vi "Main Tclk.vi"() -> ()   [LabVIEW 2018] (continued)
                w6374 = sgl 0.0 ("Single")
                n1042 = shared-variable ".\\Zeiss Library.lvlib\\Milling Z Voltage"() -> (w6355:sgl)  [unwired: 1 in, 1 out]
                "Milling Z voltage (V)" <- w6355
                n1043 = local read "FIB Options"() -> (w6358:T33)
                n1044 = local read "FIB Scan Parameters"() -> (w6356:T32)
                n1045 = local read "Milling para"() -> (w6354:T35)
                n1046 = Unbundle By Name(w6358) -> ("Flip z"=w6373:bool)
                n1047 = Unbundle By Name(w6354) -> ("FIB FOV (um)"=w6366:sgl)
                n1048 = Unbundle By Name(w6354) -> ("X size (um)"=w6352:sgl, "Line milling time (s)"=w6350:sgl, "Lines auto pause"=w6349:u16)
                n1049 = Unbundle By Name(w6356) -> ("Z size (V)"=w6357:dbl)
                n1050 = Negate(x=w6355) -> (-x=w6359:sgl)
                n1051 = Select(t=w6359, s=w6373, f=w6355) -> (s? t:f=w6360:sgl)
                n1052 = Negate(x=w6374) -> (-x=w6375:sgl)
                n1053 = Divide(x=w6360, y=w6357) -> (x/y=w6361:dbl)
                n1054 = Select(t=w6374, s=w6373, f=w6375) -> (s? t:f=w6377:sgl)
                n1055 = Multiply(x=w6361, y=w6366) -> (x*y=w6376:dbl)
                n1056 = Add(x=w6377, y=w6376) -> (x+y=w6378:dbl)
                "FIB profile Y center (um)" <- w6378
                n1057 = call "Milling parameter to trapezoidal shape.vi"("Y location (um)"=w6378, "Milling para"=w6354) -> ("X end"=w6371:dbl, "X start"=w6370:dbl, "X size (um) @ Y"=w6353:dbl)  [unwired: 5 in, 2 out]
                n1058 = expression code="x/2"(w6366) -> (w6367:sgl)
                n1059 = Add(x=w6370, y=w6371) -> (x+y=w6365:dbl)
                n1060 = Divide(x=w6353, y=w6352) -> (x/y=w6351:dbl)
                n1061 = expression code="x/2-30"(w6353) -> (w6363:dbl)
                n1062 = expression code="x/2"(w6365) -> (w6368:dbl)
                n1063 = Compound Arithmetic op=MULTIPLY(w6351, w6350, w6349) -> (→"Milling time (s)":dbl)
                n1064 = Random Number (0-1)() -> (number: 0 to 1=w6362:dbl)
                n1065 = Random Number (0-1)() -> (number: 0 to 1=w6344:dbl)
                n1066 = expression code="(x*2-1)*10"(w6362) -> (w6347:dbl)
                n1067 = Multiply(x=w6367, y=w6368) -> (x*y=w6369:dbl)
                n1068 = In Range and Coerce(upper limit=w6367, x=w6363, lower limit=0.0) -> (coerced(x)=w6346:dbl)  [unwired: 1 out]
                n1069 = Greater?(x=0.5, y=w6344) -> (0:w6342:bool)
                n1070 = Add(x=w6347, y=w6346) -> (x+y=w6345:dbl)
                n1071 = Select(t=1.0 ("f"), s=w6342, f=-1.0) -> (s? t:f=w6339:dbl)
                n1072 = Multiply(x=w6339, y=w6345) -> (x*y=w6338:dbl)
                n1073 = Add(x=w6338, y=w6369) -> (x+y=→"FIB profile X center (um)":dbl)
              }
              frame #9 {
                n1074 = local read "Re-engage counts"() -> (w6387:u8)
                n1075 = local read "Last re-engage count"() -> (w6386:u8)
                n1076 = local read "Low Mag SEM"() -> (w6395:T30)
                n1077 = local read "FIB slice #"() -> (w6393:u32)
                n1078 = local read "Milling para"() -> (w6394:T35)
                n1079 = Unbundle By Name(w6395) -> ("Low mag scan"=w6398:bool, "Prior to main scan"=w6391:bool, "Low mag interval"=w6397:u32)
                n1080 = Select(t=u32 0, s=w6391, f=u32 1 ("t")) -> (s? t:f=w6390:u32)
                n1081 = Unbundle By Name(w6394) -> ("Auto Profile"=w6379:bool)
                n1082 = Subtract(x=w6393, y=w6390) -> (x-y=w6392:u32)
                n1083 = Equal?(x=w6387, y=w6386) -> (x = y?=w6384:bool)
                n1084 = Not Equal To 0?(x=w6386) -> (x != 0?=w6385:bool)
                n1085 = Quotient & Remainder(x=w6392, y=w6397) -> (x-y*floor(x/y)=w6400:u32)  [unwired: 1 out]
                n1086 = And(x=w6384, y=w6385) -> (x .and. y?=w6382:bool)
                n1087 = local read "FIB"() -> (w6396:bool)
                n1088 = Equal To 0?(x=w6400) -> (x = 0?=w6399:bool)
                n1089 = Compound Arithmetic op=AND(w6396, w6398, w6399) -> (w6383:bool)
                n1090 = Or(x=w6382, y=w6383) -> (x .or. y?=w6381:bool)
                n1091 = And(x=w6381, y=w6379) -> (x .and. y?=w6380:bool)
                n1092 = case shown="False" w6380 {
                  frame False {
                  }
                  frame True {
                    n1093 = stacked-sequence {
                      frame #0 {
                        n1094 = local write "FIB Profile"(TRUE ("FIB Profile")) -> ()
                        n1095 = local write "Enable logging"(FALSE ("Enable logging")) -> ()
                        n1096 = Wait (ms)(milliseconds to wait=u32 200) -> ()  [unwired: 1 out]
                      }
                      frame #1 {
                        n1097 = local read "Machine Type"() -> (w6404:u8)
                        n1098 = case shown="2" w6404 {
                          frame 0, Default {
                            w6406 = sgl 90.0 ("UL-Ang")
                            n1099 = local read "FIB profile X center (um)"() -> (w6408:dbl)
                            n1100 = local read "FIB profile Y center (um)"() -> (w6409:dbl)
                            n1101 = local read "HV Data Output"() -> (w6407:T18)
                            n1102 = local read "FIB HW Config"() -> (w6416:T23)
                            n1103 = local read "FIB Options"() -> (w6417:T33)
                            n1104 = local read "Milling para"() -> (w6413:T35)
                            n1105 = local read "FIB Scan Parameters"() -> (w6414:T32)
                            n1106 = local read "Parameter Names"() -> (w6420:string[])
                            n1107 = Bundle By Name(cluster=w6414, "Frame line rampdown ratio"=0.0, "Oversampling"=u16 5) -> (w6418:T32)
                            n1108 = Bundle By Name(cluster=w6413, "X size (um)"=sgl 0.1, "Z size (um)"=sgl 10.0 ("Y size (um)"), "X center (um)"=w6408, "Z center (um)"=w6409, "UL-Ang"=w6406, "UR-Ang"=w6406) -> (w6412:T35)
                            n1109 = local read "Active logging channels"() -> (w6419:string)
                            n1110 = local write "Status message"("Scanning FIB vertically to obtain beam profile" ("Status message")) -> ()
                            n1111 = local read "Api"() -> (w6405:refnum<k7>)
                            n1112 = call "FIB profile.vi"("ActiveX Container"=w6405, "HV Data Output"=w6407, "Parameter Names"=w6420, "Active logging channels"=w6419, "Scan Para"=w6418, "Milling para"=w6412, "Options"=w6417, "HW Config"=w6416) -> ("Measurements"=w6422:dbl[][])  [unwired: 1 in, 2 out]
                            n1113 = local write "Measurements"(w6422) -> ()
                          }
                          frame 2 {
                            w6425 = sgl 90.0 ("UL-Ang")
                            n1114 = local read "FIB profile X center (um)"() -> (w6427:dbl)
                            n1115 = local read "FIB profile Y center (um)"() -> (w6428:dbl)
                            n1116 = local read "FIB HW Config"() -> (w6435:T23)
                            n1117 = local read "FIB Options"() -> (w6436:T33)
                            n1118 = local read "Milling para"() -> (w6432:T35)
                            n1119 = local read "FIB Scan Parameters"() -> (w6433:T32)
                            n1120 = local read "Parameter Names"() -> (w6439:string[])
                            n1121 = local read "Capella HV Data Output"() -> (w6426:T17)
                            n1122 = Bundle By Name(cluster=w6433, "Frame line rampdown ratio"=0.0, "Oversampling"=u16 5) -> (w6437:T32)
                            n1123 = local read "Active logging channels"() -> (w6438:string)
                            n1124 = Bundle By Name(cluster=w6432, "X size (um)"=sgl 0.1, "Z size (um)"=sgl 10.0 ("Y size (um)"), "X center (um)"=w6427, "Z center (um)"=w6428, "UL-Ang"=w6425, "UR-Ang"=w6425) -> (w6431:T35)
                            n1125 = local write "Status message"("Scanning FIB vertically to obtain beam profile" ("Status message")) -> ()
                            n1126 = local read "Api"() -> (w6424:refnum<k7>)
                            n1127 = call "FIB profile.vi"("ActiveX Container"=w6424, "Capella HV Data Output"=w6426, "Parameter Names"=w6439, "Active logging channels"=w6438, "Scan Para"=w6437, "Milling para"=w6431, "Options"=w6436, "HW Config"=w6435) -> ("Measurements"=w6441:dbl[][])  [unwired: 1 in, 2 out]
                            n1128 = local write "Measurements"(w6441) -> ()
                          }
                        }
                      }
                      frame #2 {
                        n1129 = local write "FIB Profile"(FALSE ("FIB Profile")) -> ()
                        n1130 = local write "Enable logging"(TRUE ("Enable logging")) -> ()
                      }
                    }
                  }
                }
              }
              frame #10 {
                n1131 = local read "FIB"() -> (w6445:bool)
                n1132 = case shown="True" w6445 {
                  frame False {
                  }
                  frame True {
                    n1133 = local read "Hardware Configuration"() -> (w6453:T25)
                    n1134 = Unbundle By Name(w6453) -> ("Shutter Drive"=w6452:tag)
                    n1135 = local read "Damping"() -> (w6446:bool)
                    n1136 = call "Shutter Swing V3.vi"("Shutter Drive"=w6452, "Damping"=w6446, "Shutter close"=FALSE) -> ("Shutter close fdbk"=w6449:bool, "Fail #"=w6447:u8, "SEM shutter status"=w6450:string)  [unwired: 2 in, 4 out]
                    n1137 = Greater Than 0?(x=w6447) -> (x > 0?=→"SEM shutter failed active":bool)
                    n1138 = local write "SEM shutter status"(w6450) -> ()
                    n1139 = local write "Fail #"(w6447) -> ()
                    n1140 = local write "SEM Shutter"(w6449) -> ()
                  }
                }
              }
              frame #11 {
                n1141 = local read "Low Mag SEM"() -> (w6456:T30)
                n1142 = local read "FIB slice #"() -> (w6455:u32)
                n1143 = Unbundle By Name(w6456) -> ("Low mag scan"=w6459:bool, "Prior to main scan"=w6458:bool, "Low mag interval"=w6454:u32)
                n1144 = Quotient & Remainder(x=w6455, y=w6454) -> (x-y*floor(x/y)=w6461:u32)  [unwired: 1 out]
                n1145 = local read "FIB"() -> (w6457:bool)
                n1146 = Equal To 0?(x=w6461) -> (x = 0?=w6460:bool)
                n1147 = Compound Arithmetic op=AND(w6457, w6459, w6458, w6460) -> (w6462:bool)
                n1148 = case shown="True" w6462 {
                  frame False {
                    n1149 = local write "Low Mag SEM on"(FALSE ("Mid Mag SEM on")) -> ()
                    n1150 = local write "LM overhead"(u32 0 ("LM overhead")) -> ()
                  }
                  frame True {
                    n1151 = stacked-sequence {
                      seq-local: [w6468 _] -> [_ w6480]
                      frame #0 {
                        n1152 = local read "LM SEM scan time"() -> (w6467:dbl)
                        n1153 = local read "Tiled scan inputs"() -> (w6469:T6)
                        n1154 = local read "SEM HW Config"() -> (w6470:T9)
                        n1155 = local read "Detector Information"() -> (w6471:T8)
                        n1156 = local read "SEM Scan Parameters"() -> (w6472:T26)
                        n1157 = local read "SEM Options"() -> (w6473:T27)
                        n1158 = local read "Focus Index Options"() -> (w6465:T28)
                        n1159 = local read "File Information"() -> (w6474:T31)
                        n1160 = local read "Milling para"() -> (w6475:T35)
                        n1161 = Bundle By Name(cluster=w6469, "HW Config"=w6470, "Det Info"=w6471, "SEM Scan Parameters"=w6472, "SEM Options"=w6473, "Focus Index Options"=w6465, "File Information"=w6474, "Milling para"=w6475) -> (w6468:T6)
                        n1162 = expression code="x+10"(w6467) -> (w6466:dbl)
                        n1163 = local write "LM overhead"(w6466) -> ()
                      }
                      frame #1 {
                        w6481 = FALSE ("GetInfo")
                        n1164 = local read "SEM Low Mag Scan Parameters"() -> (w6483:T5)
                        n1165 = local read "File Information"() -> (w6484:T31)
                        n1166 = Unbundle By Name(w6484) -> ("File path"=w6486:path)
                        n1167 = local write "Status message"("SEM Low Mag Scan" ("Status message")) -> ()
                        n1168 = Build Path(base path=w6486, name or relative path="Low Mag Scans\\") -> (appended path=w6487:path)
                        n1169 = local read "Api"() -> (w6476:refnum<k7>)
                        n1170 = Bundle By Name(cluster=w6480, "SEM Options.GetInfo"=w6481, "SEM Options.PNG only"=TRUE ("PNG only"), "SEM Options.Upload"=w6481, "SEM Scan Parameters"=w6483, "File Information.File path"=w6487) -> (w6477:T6)
                        n1171 = local read "WatchDog Mode"() -> (w6478:u16)
                        n1172 = call "2D scan tiled.vi"("WatchDog Mode"=w6478, "Tiled scan inputs"=w6477, "ActiveX Container"=w6476) -> ()  [unwired: 3 in, 6 out]
                        "Low Mag SEM on" <- TRUE ("Mid Mag SEM on")
                      }
                    }
                  }
                }
              }
              frame #12 {
                n1173 = local read "Mid Mag SEM"() -> (w6500:T29)
                n1174 = local read "FIB slice #"() -> (w6499:u32)
                n1175 = Subtract(x=w6499, y=u32 2) -> (x-y=w6490:u32)
                n1176 = Unbundle By Name(w6500) -> ("Mid mag scan"=w6497:bool, "Prior to main scan"=w6504:bool, "Mid mag interval"=w6489:u32)
                n1177 = Equal?(x=u32 1 ("y"), y=w6489) -> (x = y?=w6491:bool)
                n1178 = case shown="False" w6491 {
                  tunnel: [w6508 w6511] -> w6496
                  tunnel: [w6507 w6511] -> w6495
                  tunnel: [w6505 w6511] -> w6493
                  frame False {
                    n1179 = local read "Auto Focus"() -> (w6510:bool)
                    n1180 = local read "Auto Stig"() -> (w6509:bool)
                    n1181 = local read "Auto Align"() -> (w6506:bool)
                    n1182 = Not(x=w6510) -> (.not. x?=w6507:bool)
                    n1183 = Not(x=w6509) -> (.not. x?=w6508:bool)
                    n1184 = Not(x=w6506) -> (.not. x?=w6505:bool)
                  }
                  frame True {
                    w6511 = TRUE
                  }
                }
                n1185 = Quotient & Remainder(x=w6490, y=w6489) -> (x-y*floor(x/y)=w6502:u32)  [unwired: 1 out]
                n1186 = local read "FIB"() -> (w6498:bool)
                n1187 = Equal To 0?(x=w6502) -> (x = 0?=w6503:bool)
                n1188 = Compound Arithmetic op=AND(w6498, w6495, w6496, w6493, w6497, w6504, w6503) -> (w6501:bool)
                n1189 = case shown="True" w6501 {
                  frame False {
                    n1190 = local write "Mid Mag SEM on"(FALSE ("Mid Mag SEM on")) -> ()
                    n1191 = local write "MM overhead"(u32 0 ("MM overhead")) -> ()
                  }
                  frame True {
                    n1192 = stacked-sequence {
                      seq-local: [w6517 _] -> [_ w6528]
                      frame #0 {
                        n1193 = local read "Tiled scan inputs"() -> (w6518:T6)
                        n1194 = local read "SEM HW Config"() -> (w6519:T9)
                        n1195 = local read "Detector Information"() -> (w6520:T8)
                        n1196 = local read "SEM Scan Parameters"() -> (w6521:T26)
                        n1197 = local read "SEM Options"() -> (w6522:T27)
                        n1198 = local read "Focus Index Options"() -> (w6514:T28)
                        n1199 = local read "File Information"() -> (w6523:T31)
                        n1200 = local read "MM SEM scan time"() -> (w6515:dbl)
                        n1201 = local read "Milling para"() -> (w6524:T35)
                        n1202 = Bundle By Name(cluster=w6518, "HW Config"=w6519, "Det Info"=w6520, "SEM Scan Parameters"=w6521, "SEM Options"=w6522, "Focus Index Options"=w6514, "File Information"=w6523, "Milling para"=w6524) -> (w6517:T6)
                        n1203 = expression code="x+10"(w6515) -> (w6516:dbl)
                        n1204 = local write "MM overhead"(w6516) -> ()
                      }
                      frame #1 {
                        w6534 = FALSE ("GetInfo")
                        n1205 = local read "SEM Mid Mag Scan Parameters"() -> (w6533:T5)
                        n1206 = local read "File Information"() -> (w6532:T31)
                        n1207 = Unbundle By Name(w6532) -> ("File path"=w6530:path)
                        n1208 = local write "Status message"("SEM Mid Mag Scan" ("Status message")) -> ()
                        n1209 = Build Path(base path=w6530, name or relative path="Mid Mag Scans\\") -> (appended path=w6529:path)
                        n1210 = local read "Api"() -> (w6525:refnum<k7>)
                        n1211 = Bundle By Name(cluster=w6528, "SEM Options.GetInfo"=w6534, "SEM Options.PNG only"=w6534, "SEM Options.Upload"=w6534, "SEM Scan Parameters"=w6533, "File Information.File path"=w6529) -> (w6526:T6)
                        n1212 = local read "WatchDog Mode"() -> (w6527:u16)
                        n1213 = call "2D scan tiled.vi"("WatchDog Mode"=w6527, "Tiled scan inputs"=w6526, "ActiveX Container"=w6525) -> ()  [unwired: 3 in, 6 out]
                        "Mid Mag SEM on" <- TRUE ("Mid Mag SEM on")
                      }
                    }
                  }
                }
              }
              frame #13 {
                n1214 = local read "Auto re-engage"() -> (w6537:bool)
                n1215 = case shown="True" w6537 {
                  frame False {
                    n1216 = local read "Auto Align"() -> (w6539:bool)
                    n1217 = local read "Auto Focus"() -> (w6541:bool)
                    n1218 = local read "Auto Stig"() -> (w6540:bool)
                    n1219 = local read "Re-engage counts"() -> (w6545:u8)
                    n1220 = local read "Last re-engage count"() -> (w6544:u8)
                    n1221 = Build Array(w6541, w6540, w6539) -> (w6542:bool[])
                    n1222 = Equal?(x=w6545, y=w6544) -> (x = y?=w6543:bool)
                    n1223 = Boolean Array To Number(Boolean array=w6542) -> (number=w6538:u32)
                    n1224 = case shown="6" w6538 {
                      frame 0, Default {
                      }
                      frame 3 {
                        n1225 = local write "Auto Stig"(FALSE ("Auto Focus")) -> ()
                      }
                      frame 5 {
                        n1226 = local write "Auto Align"(FALSE ("Auto Focus")) -> ()
                      }
                      frame 6 {
                        n1227 = local write "Auto Align"(FALSE ("Auto Focus")) -> ()
                      }
                      frame 7 {
                        w6550 = FALSE ("Auto Focus")
                        n1228 = local write "Auto Stig"(w6550) -> ()
                        n1229 = local write "Auto Align"(w6550) -> ()
                      }
                    }
                    n1230 = case shown="False" w6543 {
                      tunnel: [w6552 w6553] -> w6546
                      tunnel: w6545 -> [w6551 _]
                      frame False {
                        n1231 = Increment(x=w6551) -> (x+1=w6552:u8)
                      }
                      frame True {
                        w6553 = u8 0
                        n1232 = local write "Last re-engage count"(w6553) -> ()
                      }
                    }
                    n1233 = local write "Re-engage counts"(w6546) -> ()
                  }
                  frame True {
                    w6556 = T44."Enabled" ("Disabled")
                    w6557 = T44."Disabled and Grayed Out" ("Disabled")
                    w6558 = u8 0 ("AF Count")
                    w6555 = 0.0 ("f")
                    w6560 = FALSE ("Auto Focus")
                    n1234 = local write "Auto Focus"(w6560) -> ()
                    n1235 = local write "Auto Stig"(w6560) -> ()
                    n1236 = local write "Auto Align"(w6560) -> ()
                    n1237 = local read "Focus Index"() -> (w6590:sgl)
                    n1238 = local read "Pre-reheat FI"() -> (w6591:dbl)
                    n1239 = local read "Pre-reheat X center (um)"() -> (w6577:dbl)
                    n1240 = local read "Re-engage X shift (um)"() -> (w6565:dbl)
                    n1241 = local read "Pre-reheat Y center (um)"() -> (w6592:dbl)
                    n1242 = local read "Re-engage Y shift (um)"() -> (w6568:dbl)
                    n1243 = local read "Pre-reheat Y stig"() -> (w6559:sgl[][])
                    n1244 = local read "FIB-SEM Angle"() -> (w6562:dbl)
                    n1245 = expression code="x*0.9"(w6591) -> (w6589:dbl)
                    n1246 = expression code="cos(x*pi/180)"(w6562) -> (w6561:dbl)
                    n1247 = local write "AF Count"(w6558) -> ()
                    n1248 = local write "AS Count"(w6558) -> ()
                    n1249 = local write "AA Count"(w6558) -> ()
                    n1250 = local read "Re-engage counts"() -> (w6570:u8)
                    n1251 = local read "Recovered counts"() -> (w6583:u8)
                    n1252 = local write "Re-engage cancelled"("Cancel Auto re-engage") -> ()
                    n1253 = Greater Or Equal?(x=w6590, y=w6589) -> (x >= y?=w6587:bool)
                    n1254 = Power Of X(1:w6568, 2:"b") -> (0:w6574:dbl)
                    n1255 = Select(t=u8 1, s=w6587, f=u8 0) -> (s? t:f=w6584:u8)
                    n1256 = Compound Arithmetic op=MULTIPLY(w6574, "a", w6561) -> (w6572:dbl)
                    "Re-engage Y stig shift" <- w6572
                    n1257 = Increment(x=w6570) -> (x+1=w6569:u8)
                    n1258 = Add(x=w6584, y=w6583) -> (x+y=w6571:u8)
                    n1259 = Not(x="Cancel Auto re-engage") -> (.not. x?=w6588:bool)
                    n1260 = local write "Re-engage counts"(w6569) -> ()
                    n1261 = Less Or Equal?(x=w6571, y=u8 11) -> (x <= y?=w6581:bool)
                    n1262 = local write "Recovered counts"(w6571) -> ()
                    n1263 = And(x=w6581, y=w6588) -> (x .and. y?=w6579:bool)
                    n1264 = Select(t=w6565, s=w6579, f=w6555) -> (s? t:f=w6578:dbl)
                    n1265 = Select(t=w6568, s=w6579, f=w6555) -> (s? t:f=w6580:dbl)
                    n1266 = Select(t=w6572, s=w6579, f=w6555) -> ()  [unwired: 1 out]
                    n1267 = Add(x=w6577, y=w6578) -> (x+y=w6576:dbl)
                    n1268 = Add(x=w6592, y=w6580) -> (x+y=w6595:dbl)
                    n1269 = Add(x=w6559, y=w6555) -> (x+y=w6593:dbl[][])
                    n1270 = local write "Auto re-engage"(w6579) -> ()
                    n1271 = case shown="False" w6579 {
                      tunnel: w6569 -> [w6600 _]
                      frame False {
                        w6597 = T44."Enabled" ("Disabled")
                        n1272 = Increment(x=w6600) -> (x+1=w6599:u8)
                        n1273 = local read "Prior Alert Settings"() -> (w6598:T2)
                        n1274 = local write "Last re-engage count"(w6599) -> ()
                        n1275 = local write "Recovered counts"(u8 0 ("Recovered counts")) -> ()
                        n1276 = property on="Pause for reheat" class="Bool (strict)"("DisabledEnum"=T44."Enabled" ("Disabled")) -> ()  [unwired: 2 in, 2 out]
                        n1277 = local write "Alert Settings"(w6598) -> ()
                        n1278 = local write "Cancel Auto re-engage"(FALSE ("Cancel Auto re-engage")) -> ()
                        n1279 = property on="Auto Focus" class="Bool (strict)"("DisabledEnum"=w6597) -> ()  [unwired: 2 in, 2 out]
                        n1280 = property on="Auto Stig" class="Bool (strict)"("DisabledEnum"=w6597) -> ()  [unwired: 2 in, 2 out]
                        n1281 = property on="Auto Align" class="Bool (strict)"("DisabledEnum"=w6597) -> ()  [unwired: 2 in, 2 out]
                      }
                      frame True {
                      }
                    }
                    n1282 = local read "SEM Scan Parameters"() -> (w6596:T26)
                    n1283 = Bundle By Name(cluster=w6596, "X center (um)"=w6576, "Y center (um)"=w6595, "Y stig"=w6593) -> (w6594:T26)
                    n1284 = local write "SEM Scan Parameters"(w6594) -> ()
                    n1285 = property on="Auto Focus" class="Bool (strict)"("DisabledEnum"=w6557) -> ()  [unwired: 2 in, 2 out]
                    n1286 = property on="Auto Stig" class="Bool (strict)"("DisabledEnum"=w6557) -> ()  [unwired: 2 in, 2 out]
                    n1287 = property on="Auto Align" class="Bool (strict)"("DisabledEnum"=w6557) -> ()  [unwired: 2 in, 2 out]
                    n1288 = local read "Re-engage X shift array"() -> (w6564:dbl[])
                    n1289 = local read "Re-engage Y shift array"() -> (w6567:dbl[])
                    n1290 = property on="AF Steps" class="DigNum (strict)"("DisabledEnum"=w6556) -> ()  [unwired: 2 in, 2 out]
                    n1291 = property on="AS Steps" class="DigNum (strict)"("DisabledEnum"=w6556) -> ()  [unwired: 2 in, 2 out]
                    n1292 = property on="AA Steps" class="DigNum (strict)"("DisabledEnum"=w6556) -> ()  [unwired: 2 in, 2 out]
                    n1293 = Build Array (concatenate)(w6564, w6565) -> (w6563:dbl[])
                    n1294 = Build Array (concatenate)(w6567, w6568) -> (w6566:dbl[])
                    n1295 = local write "Re-engage X shift array"(w6563) -> ()
                    n1296 = local write "Re-engage Y shift array"(w6566) -> ()
                  }
                }
              }
              frame #14 {
                n1297 = case shown="False" "Auto Focus" {
                  frame False {
                    n1298 = local read "WD array tiled"() -> (w6606:sgl[][][])
                    n1299 = local read "Auto Stig"() -> (w6611:bool)
                    n1300 = local read "Auto Align"() -> (w6610:bool)
                    n1301 = Not(x=w6611) -> (.not. x?=w6608:bool)
                    n1302 = Not(x=w6610) -> (.not. x?=w6607:bool)
                    n1303 = Empty Array?(array=w6606) -> (empty?=w6605:bool)
                    n1304 = Compound Arithmetic op=AND(w6605, w6608, w6607) -> (w6609:bool)
                    n1305 = case shown="False" w6605 {
                      frame False {
                        n1306 = property on="Auto Focus" class="Bool (strict)"("DisabledEnum"=T44."Disabled and Grayed Out" ("Disabled")) -> ()  [unwired: 2 in, 2 out]
                      }
                      frame True {
                      }
                    }
                    n1307 = case shown="True" w6609 {
                      frame False {
                      }
                      frame True {
                        w6612 = T44."Enabled" ("Disabled")
                        n1308 = property on="Auto Stig" class="Bool (strict)"("DisabledEnum"=w6612) -> ()  [unwired: 2 in, 2 out]
                        n1309 = property on="Auto Align" class="Bool (strict)"("DisabledEnum"=w6612) -> ()  [unwired: 2 in, 2 out]
                      }
                    }
                  }
                  frame True {
                    w6623 = T44."Disabled and Grayed Out" ("Disabled")
                    n1310 = local read "SEM Scan Parameters"() -> (w6621:T26)
                    n1311 = local read "AF Count"() -> (w6618:u8)
                    n1312 = Increment(x=w6618) -> (x+1=w6622:u8)
                    n1313 = Equal To 0?(x=w6618) -> (x = 0?=w6617:bool)
                    n1314 = local write "AF Count"(w6622) -> ()
                    n1315 = property on="Auto Stig" class="Bool (strict)"("DisabledEnum"=w6623) -> ()  [unwired: 2 in, 2 out]
                    n1316 = property on="X Grids" class="Arr (strict)"("DisabledEnum"=w6623) -> ()  [unwired: 2 in, 2 out]
                    n1317 = property on="Primary X index" class="Arr (strict)"("DisabledEnum"=w6623) -> ()  [unwired: 2 in, 2 out]
                    n1318 = Unbundle By Name(w6621) -> ("Y tiles"=w6620:u8, "X tiles"=w6619:u8)
                    n1319 = property on="Auto Align" class="Bool (strict)"("DisabledEnum"=w6623) -> ()  [unwired: 2 in, 2 out]
                    n1320 = case shown="True" w6617 {
                      tunnel: w6620 -> [_ w6629]
                      tunnel: w6619 -> [_ w6630]
                      frame False {
                      }
                      frame True {
                        n1321 = Initialize Array(FALSE ("ASX Success"), w6629, w6630) -> (w6634:bool[][])
                        n1322 = Initialize Array(u8 0 ("Skip Steps"), w6629, w6630) -> (w6631:u8[][])
                        n1323 = local write "Skip Steps tiled"(w6631) -> ()
                        n1324 = local write "AF Success tiled"(w6634) -> ()
                        n1325 = local write "Image Tabs"(T37."Auto Focus / Stig / Align" ("Image Tabs")) -> ()
                      }
                    }
                    n1326 = property on="Y Grids" class="Arr (strict)"("DisabledEnum"=w6623) -> ()  [unwired: 2 in, 2 out]
                    n1327 = property on="Primary Y index" class="Arr (strict)"("DisabledEnum"=w6623) -> ()  [unwired: 2 in, 2 out]
                    n1328 = property on="Keep aspect ratio" class="Bool (strict)"("DisabledEnum"=w6623) -> ()  [unwired: 2 in, 2 out]
                    n1329 = local read "Focus Index Options"() -> (w6616:T28)
                    n1330 = Unbundle By Name(w6616) -> ("Y Grids"=w6615:u8[][])
                    n1331 = Array Max & Min(array=w6615) -> (max value=w6614:u8)  [unwired: 3 out]
                    n1332 = Greater Or Equal?(x=w6614, y=u8 2) -> (x >= y?=w6627:bool)
                    n1333 = Select(t=T44."Enabled" ("Disabled"), s=w6627, f=T44."Disabled and Grayed Out" ("Disabled")) -> (s? t:f=w6624:T44)
                    n1334 = property on="Slope tiled" class="Arr (strict)"("DisabledEnum"=w6624) -> ()  [unwired: 2 in, 2 out]
                    n1335 = property on="Dynamic Focus" class="XYGraph (strict)"("DisabledEnum"=w6624) -> ()  [unwired: 2 in, 2 out]
                  }
                }
              }
              frame #15 {
                n1336 = case shown="False" "Auto Stig" {
                  frame False {
                    n1337 = local read "StigX array tiled"() -> (w6672:sgl[][][])
                    n1338 = local read "StigY array tiled"() -> (w6673:sgl[][][])
                    n1339 = local read "Auto Focus"() -> (w6676:bool)
                    n1340 = local read "Auto Align"() -> (w6677:bool)
                    n1341 = Empty Array?(array=w6672) -> (empty?=w6671:bool)
                    n1342 = Empty Array?(array=w6673) -> (empty?=w6670:bool)
                    n1343 = local write "Stig Options"(enum16{"Defaut", "Stig X", "Stig Y"}."Defaut" ("Stig Options")) -> ()
                    n1344 = Not(x=w6676) -> (.not. x?=w6678:bool)
                    n1345 = Not(x=w6677) -> (.not. x?=w6679:bool)
                    n1346 = And(x=w6671, y=w6670) -> (x .and. y?=w6674:bool)
                    n1347 = Compound Arithmetic op=AND(w6674, w6678, w6679) -> (w6675:bool)
                    n1348 = case shown="False" w6674 {
                      frame False {
                        n1349 = property on="Auto Stig" class="Bool (strict)"("DisabledEnum"=T44."Disabled and Grayed Out" ("Disabled")) -> ()  [unwired: 2 in, 2 out]
                      }
                      frame True {
                      }
                    }
                    n1350 = case shown="True" w6675 {
                      frame False {
                      }
                      frame True {
                        w6681 = T44."Enabled" ("Disabled")
                        n1351 = property on="Auto Focus" class="Bool (strict)"("DisabledEnum"=w6681) -> ()  [unwired: 2 in, 2 out]
                        n1352 = property on="Auto Align" class="Bool (strict)"("DisabledEnum"=w6681) -> ()  [unwired: 2 in, 2 out]
                      }
                    }
                  }
                  frame True {
                    w6689 = T44."Disabled and Grayed Out" ("Disabled")
                    n1353 = local read "SEM Scan Parameters"() -> (w6687:T26)
                    n1354 = local read "AS Count"() -> (w6684:u8)
                    n1355 = local read "Stig Options"() -> (w6693:enum16{"Defaut", "Stig X", "Stig Y"})
                    n1356 = Increment(x=w6684) -> (x+1=w6688:u8)
                    n1357 = Equal To 0?(x=w6684) -> (x = 0?=w6683:bool)
                    n1358 = local write "AS Count"(w6688) -> ()
                    n1359 = Unbundle By Name(w6687) -> ("Y tiles"=w6686:u8, "X tiles"=w6685:u8)
                    n1360 = Equal?(x=w6693, y=enum16{"Defaut", "Stig X", "Stig Y"}."Defaut" ("Stig Options")) -> (x = y?=w6690:bool)
                    n1361 = property on="Auto Focus" class="Bool (strict)"("DisabledEnum"=w6689) -> ()  [unwired: 2 in, 2 out]
                    n1362 = And(x=w6683, y=w6690) -> (x .and. y?=w6691:bool)
                    n1363 = case shown="True" w6691 {
                      tunnel: w6686 -> [_ w6696]
                      tunnel: w6685 -> [_ w6695]
                      frame False {
                      }
                      frame True {
                        n1364 = Initialize Array(FALSE ("ASX Success"), w6696, w6695) -> (w6699:bool[][])
                        n1365 = Initialize Array(u8 0 ("Skip Steps"), w6696, w6695) -> (w6694:u8[][])
                        n1366 = local write "ASX Success tiled"(w6699) -> ()
                        n1367 = local write "ASY Success tiled"(w6699) -> ()
                        n1368 = local write "Skip Steps tiled"(w6694) -> ()
                        n1369 = local write "Stig Options"(enum16{"Defaut", "Stig X", "Stig Y"}."Stig X" ("Stig Options")) -> ()
                        n1370 = local write "Image Tabs"(T37."Auto Focus / Stig / Align" ("Image Tabs")) -> ()
                      }
                    }
                    n1371 = property on="Auto Align" class="Bool (strict)"("DisabledEnum"=w6689) -> ()  [unwired: 2 in, 2 out]
                  }
                }
                n1372 = case shown="True" "Auto Align" {
                  frame False {
                    n1373 = local read "AlnX array tiled"() -> (w6640:sgl[][][])
                    n1374 = local read "AlnY array tiled"() -> (w6641:sgl[][][])
                    n1375 = local read "Auto Focus"() -> (w6645:bool)
                    n1376 = local read "Auto Stig"() -> (w6646:bool)
                    n1377 = Empty Array?(array=w6640) -> (empty?=w6639:bool)
                    n1378 = Empty Array?(array=w6641) -> (empty?=w6638:bool)
                    n1379 = local write "Aln Options"(enum16{"Defaut", "Aln X", "Aln Y"}."Defaut" ("Stig Options")) -> ()
                    n1380 = Not(x=w6645) -> (.not. x?=w6647:bool)
                    n1381 = Not(x=w6646) -> (.not. x?=w6648:bool)
                    n1382 = And(x=w6639, y=w6638) -> (x .and. y?=w6643:bool)
                    n1383 = Compound Arithmetic op=AND(w6643, w6647, w6648) -> (w6644:bool)
                    n1384 = case shown="False" w6643 {
                      frame False {
                        n1385 = property on="Auto Align" class="Bool (strict)"("DisabledEnum"=T44."Disabled and Grayed Out" ("Disabled")) -> ()  [unwired: 2 in, 2 out]
                      }
                      frame True {
                      }
                    }
                    n1386 = case shown="True" w6644 {
                      frame False {
                      }
                      frame True {
                        w6649 = T44."Enabled" ("Disabled")
                        n1387 = property on="Auto Focus" class="Bool (strict)"("DisabledEnum"=w6649) -> ()  [unwired: 2 in, 2 out]
                        n1388 = property on="Auto Stig" class="Bool (strict)"("DisabledEnum"=w6649) -> ()  [unwired: 2 in, 2 out]
                      }
                    }
                  }
                  frame True {
                    w6653 = T44."Disabled and Grayed Out" ("Disabled")
                    n1389 = local read "SEM Scan Parameters"() -> (w6657:T26)
                    n1390 = local read "AA Count"() -> (w6652:u8)
                    n1391 = local read "Aln Options"() -> (w6661:enum16{"Defaut", "Aln X", "Aln Y"})
                    n1392 = Increment(x=w6652) -> (x+1=w6658:u8)
                    n1393 = Equal To 0?(x=w6652) -> (x = 0?=w6651:bool)
                    n1394 = local write "AA Count"(w6658) -> ()
                    n1395 = Unbundle By Name(w6657) -> ("Y tiles"=w6656:u8, "X tiles"=w6655:u8)
                    n1396 = Equal?(x=w6661, y=enum16{"Defaut", "Aln X", "Aln Y"}."Defaut" ("Aln Options")) -> (x = y?=w6659:bool)
                    n1397 = property on="Auto Focus" class="Bool (strict)"("DisabledEnum"=w6653) -> ()  [unwired: 2 in, 2 out]
                    n1398 = And(x=w6651, y=w6659) -> (x .and. y?=w6660:bool)
                    n1399 = case shown="True" w6660 {
                      tunnel: w6656 -> [_ w6665]
                      tunnel: w6655 -> [_ w6664]
                      frame False {
                      }
                      frame True {
                        n1400 = Initialize Array(FALSE ("ASX Success"), w6665, w6664) -> (w6668:bool[][])
                        n1401 = Initialize Array(u8 0 ("Skip Steps"), w6665, w6664) -> (w6663:u8[][])
                        n1402 = local write "AAX Success tiled"(w6668) -> ()
                        n1403 = local write "AAY Success tiled"(w6668) -> ()
                        n1404 = local write "Skip Steps tiled"(w6663) -> ()
                        n1405 = local write "Aln Options"(enum16{"Defaut", "Aln X", "Aln Y"}."Aln X" ("Stig Options")) -> ()
                        n1406 = local write "Image Tabs"(T37."Auto Focus / Stig / Align" ("Image Tabs")) -> ()
                      }
                    }
                    n1407 = property on="Auto Stig" class="Bool (strict)"("DisabledEnum"=w6653) -> ()  [unwired: 2 in, 2 out]
                  }
                }
              }
              frame #16 {
                w6704 = 20.0 ("upper limit")
                n1408 = local read "SEM Scan Parameters"() -> (w6728:T26)
                n1409 = local read "FIB slice #"() -> (w6736:u32)
                n1410 = local read "Machine Type"() -> (w6725:u8)
                n1411 = shared-variable "My Computer\\Zeiss Library.lvlib\\FIB Slice #"(w6736) -> ()  [unwired: 1 in, 1 out]
                n1412 = Equal To 0?(x=w6736) -> (x = 0?=w6758:bool)
                n1413 = Or(x=w6758, y="Reset Focus") -> (x .or. y?=w6730:bool)
                n1414 = local read "Milling para"() -> (w6751:T35)
                n1415 = local read "FIB-SEM Angle"() -> (w6754:dbl)
                n1416 = Unbundle By Name(w6728) -> ("X size (um)"=w6703:sgl, "Y size (um)"=w6710:sgl, "X size auto"=w6720:bool, "X size (V)"=w6717:dbl)
                n1417 = case shown="True" w6730 {
                  tunnel: [w6764 w6771] -> w6734
                  tunnel: [w6763 w6770] -> w6733
                  tunnel: [w6762 w6769] -> w6735
                  tunnel: [w6761 w6768] -> w6732
                  tunnel: [w6760 w6767] -> w6731
                  tunnel: w6728 -> [w6759 w6766]
                  tunnel: w6725 -> [_ w6765]
                  frame False {
                    n1418 = Unbundle By Name(w6759) -> ("WD (mm)"=w6762:sgl[][], "X stig"=w6764:sgl[][], "Y stig"=w6763:sgl[][], "X aln"=w6761:sgl[][], "Y aln"=w6760:sgl[][])
                  }
                  frame True {
                    n1419 = stacked-sequence {
                      tunnel: [_ w6779] -> w6771
                      tunnel: [_ w6778] -> w6770
                      tunnel: [_ w6777] -> w6769
                      tunnel: [_ w6776] -> w6768
                      tunnel: [_ w6775] -> w6767
                      tunnel: w6766 -> [_ w6774]
                      tunnel: w6765 -> [_ w6773]
                      frame #0 {
                        n1420 = local read "SEM Options"() -> (→"Initial Options":T27)
                      }
                      frame #1 {
                        n1421 = case shown="0, Default" w6773 {
                          tunnel: [w6787 w6867] -> w6779
                          tunnel: [w6786 w6866] -> w6778
                          tunnel: [w6785 w6868] -> w6777
                          tunnel: [w6784 w6865] -> w6776
                          tunnel: [w6783 w6864] -> w6775
                          tunnel: w6774 -> [w6780 _]
                          frame 0, Default {
                            n1422 = local read "Hardware Configuration"() -> (w6782:T25)
                            n1423 = Unbundle By Name(w6782) -> ("Eanable COM"=w6781:bool)
                            n1424 = case shown="True" w6781 {
                              tunnel: [w6791 w6801] -> w6787
                              tunnel: [w6790 w6800] -> w6786
                              tunnel: [w6792 w6806] -> w6785
                              tunnel: [w6789 w6799] -> w6784
                              tunnel: [w6788 w6798] -> w6783
                              tunnel: w6780 -> [w6793 _]
                              frame False {
                                n1425 = Unbundle By Name(w6793) -> ("WD (mm)"=w6792:sgl[][], "X stig"=w6791:sgl[][], "Y stig"=w6790:sgl[][], "X aln"=w6789:sgl[][], "Y aln"=w6788:sgl[][])
                              }
                              frame True {
                                w6820 = TRUE ("Initialization")
                                w6811 = 0 ("offset past token")
                                n1426 = local read "COM port"() -> (w6824:refnum<visa-resource-name>)
                                n1427 = call "Remcon32 command.vi"("Initialization"=w6820, "SEM command"="sti? " ("write buffer"), "COM port in"=w6824) -> ("error out"=w6814:errorcluster, "SEM reply"=w6821:string, "COM port out"=w6816:refnum<visa-resource-name>)  [unwired: 2 in, 4 out]
                                n1428 = while {
                                shift-right: [w6842] -> _
                                shift-left: w6811 -> [w6845]
                                tunnel: [w6843] -> w6827 mode=indexing
                                tunnel: w6821 -> [w6840]
                                stop <- w6841 stop-if-true
                                n1429 = Scan String For Tokens(8:w6845, 9:w6840) -> (1:w6843:string, 2:w6842:i32)  [unwired: 1 in, 5 out]
                                n1430 = Less?(x=w6842, y=0) -> (x < y?=w6841:bool)
                                }
                                n1431 = call "Remcon32 command.vi"("error in"=w6814, "SEM command"="aln? " ("write buffer"), "COM port in"=w6816) -> ("error out"=w6813:errorcluster, "SEM reply"=w6812:string, "COM port out"=w6815:refnum<visa-resource-name>)  [unwired: 2 in, 4 out]
                                n1432 = while {
                                shift-right: [w6833] -> _
                                shift-left: w6811 -> [w6836]
                                tunnel: [w6834] -> w6817 mode=indexing
                                tunnel: w6812 -> [w6831]
                                stop <- w6832 stop-if-true
                                n1433 = Scan String For Tokens(8:w6836, 9:w6831) -> (1:w6834:string, 2:w6833:i32)  [unwired: 1 in, 5 out]
                                n1434 = Less?(x=w6833, y=0) -> (x < y?=w6832:bool)
                                }
                                n1435 = for {
                                tunnel: w6827 -> [w6839] mode=indexing
                                tunnel: [w6838] -> w6826 mode=indexing
                                n1436 = Fract/Exp String To Number(string=w6839, default (0 dbl)=sgl 0.0 ("default (0 DBL)")) -> (number=w6838:sgl)  [unwired: 3 out]
                                }
                                n1437 = for {
                                tunnel: w6817 -> [w6830] mode=indexing
                                tunnel: [w6829] -> w6818 mode=indexing
                                n1438 = Fract/Exp String To Number(string=w6830, default (0 dbl)=sgl 0.0 ("default (0 DBL)")) -> (number=w6829:sgl)  [unwired: 3 out]
                                }
                                n1439 = call "Remcon32 command.vi"("Close session"=w6820, "error in"=w6813, "SEM command"="foc? " ("write buffer"), "COM port in"=w6815) -> ("SEM reply"=w6822:string)  [unwired: 1 in, 6 out]
                                n1440 = local read "WD Stig Aln tile offsets"() -> (w6809:T3)
                                n1441 = Fract/Exp String To Number(string=w6822, default (0 dbl)=sgl 0.0 ("default (0 DBL)")) -> (number=w6807:sgl)  [unwired: 3 out]
                                n1442 = Index Array(array=w6826) -> (element #1=w6797:sgl, element #2=w6796:sgl)  [unwired: 2 in]
                                n1443 = Index Array(array=w6818) -> (element #1=w6795:sgl, element #2=w6794:sgl)  [unwired: 2 in]
                                n1444 = Unbundle By Name(w6809) -> ("dWD"=w6808:sgl[][], "dX stig"=w6805:sgl[][], "dY stig"=w6804:sgl[][], "dX aln"=w6803:sgl[][], "dY aln"=w6802:sgl[][])
                                n1445 = Add(x=w6808, y=w6807) -> (x+y=w6806:sgl[][])
                                n1446 = Add(x=w6805, y=w6797) -> (x+y=w6801:sgl[][])
                                n1447 = Add(x=w6804, y=w6796) -> (x+y=w6800:sgl[][])
                                n1448 = Add(x=w6803, y=w6795) -> (x+y=w6799:sgl[][])
                                n1449 = Add(x=w6802, y=w6794) -> (x+y=w6798:sgl[][])
                              }
                            }
                          }
                          frame 2 {
                            n1450 = local read "Api"() -> (w6859:refnum<k7>)
                            n1451 = call "SmartSEM Remote API get float.vi"("lpszParam"="AP_WD", "ActiveX Container"=w6859) -> ("error out"=w6848:errorcluster, "vValue"=w6861:sgl)  [unwired: 7 in, 1 out]
                            n1452 = call "SmartSEM Remote API get float.vi"("error in"=w6848, "lpszParam"="AP_STIG_X", "ActiveX Container"=w6859) -> ("error out"=w6847:errorcluster, "vValue"=w6854:sgl, "reference out"=w6857:refnum<k7>)  [unwired: 6 in]
                            n1453 = expression code="x*1000"(w6861) -> (w6863:sgl)
                            n1454 = call "SmartSEM Remote API get float.vi"("error in"=w6847, "lpszParam"="AP_APERTURE_ALIGN_X", "ActiveX Container"=w6857) -> ("error out"=w6846:errorcluster, "vValue"=w6855:sgl)  [unwired: 6 in, 1 out]
                            n1455 = call "SmartSEM Remote API get float.vi"("error in"=w6846, "lpszParam"="AP_STIG_Y", "ActiveX Container"=w6859) -> ("error out"=w6852:errorcluster, "vValue"=w6849:sgl, "reference out"=w6853:refnum<k7>)  [unwired: 6 in]
                            n1456 = call "SmartSEM Remote API get float.vi"("error in"=w6852, "lpszParam"="AP_APERTURE_ALIGN_Y", "ActiveX Container"=w6853) -> ("vValue"=w6850:sgl)  [unwired: 6 in, 2 out]
                            n1457 = local read "WD Stig Aln tile offsets"() -> (w6869:T3)
                            n1458 = Unbundle By Name(w6869) -> ("dWD"=w6870:sgl[][], "dX stig"=w6871:sgl[][], "dY stig"=w6872:sgl[][], "dX aln"=w6873:sgl[][], "dY aln"=w6874:sgl[][])
                            n1459 = Add(x=w6870, y=w6863) -> (x+y=w6868:sgl[][])
                            n1460 = Add(x=w6871, y=w6854) -> (x+y=w6867:sgl[][])
                            n1461 = Add(x=w6872, y=w6849) -> (x+y=w6866:sgl[][])
                            n1462 = Add(x=w6873, y=w6855) -> (x+y=w6865:sgl[][])
                            n1463 = Add(x=w6874, y=w6850) -> (x+y=w6864:sgl[][])
                          }
                        }
                      }
                    }
                  }
                }
                n1464 = Unbundle By Name(w6728) -> ("X center (um)"=w6727:sgl, "Y center (um)"=w6726:sgl)
                n1465 = Unbundle By Name(w6751) -> ("Z-step (nm)"=w6724:dbl, "Lines auto pause"=w6723:u16)
                n1466 = expression code="cos(x/180*pi)"(w6754) -> (w6755:dbl)
                n1467 = local read "SEM FOV"() -> (w6719:dbl)
                n1468 = Divide(x=w6703, y=w6710) -> (x/y=w6711:sgl)
                n1469 = In Range and Coerce(upper limit=1.0, x=w6711, lower limit=0.001) -> (coerced(x)=w6714:dbl)  [unwired: 1 out]
                n1470 = Divide(x=w6703, y=w6719) -> (x/y=w6721:dbl)
                n1471 = Compound Arithmetic op=MULTIPLY(w6724, w6723, w6755) -> (w6750:dbl)
